vi "RPiReceive.vi"   [LabVIEW 2013]
uses:
  VisionData.ctl
types:
  T1 = typedef "VisionData.ctl" = cluster{"Total":u8, "Timestamp":u32, "Horizontal":u8, "Vertical":u8, "Left Hot":bool, "Right Hot":bool}
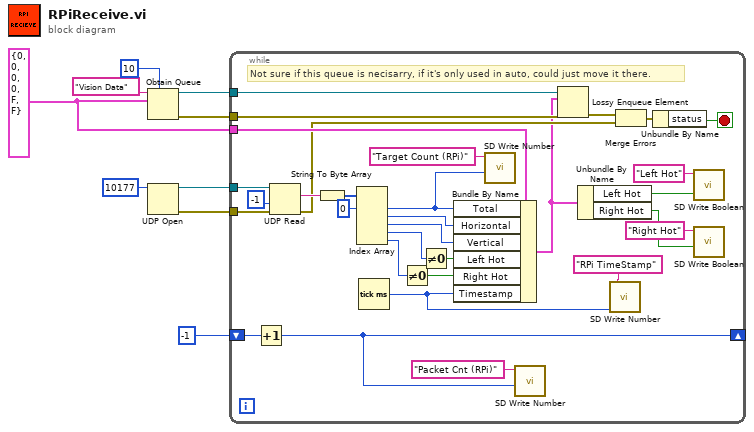
[diagram p0: block diagram]
diagram:
  w7 = T1 {"Total"=0, "Timestamp"=0, "Horizontal"=0, "Vertical"=0, "Left Hot"=FALSE, "Right Hot"=FALSE}
  n1 = Obtain Queue(max queue size (-1, unlimited)=10, name (unnamed)="Vision Data", element data type=w7) -> (queue out=w4:refnum<queue>, error out=w8:errorcluster)  [unwired: 2 in, 1 out]
  n2 = UDP Open(11:u16 10177 ("port")) -> (port=w2:refnum<k16>, 0:w3:errorcluster)  [unwired: 4 in, 1 out]
  n3 = while {
    tunnel: w2 -> [w40]
    tunnel: w3 -> [w39]
    tunnel: w4 -> [w35]
    tunnel: w7 -> [w34]
    tunnel: w8 -> [w33]
    shift-right: [w25] -> _
    shift-left: -1 -> [w24]
    stop <- w29 stop-if-true
    # "Not sure if this queue is necisarry, if it's only used in auto, could just move it there."
    n4 = Increment(x=w24) -> (x+1=w25:i32)
    n5 = UDP Read(connection ID=w40, timeout ms (25000)=-1, 8:w39) -> (data out=w37:string, error out=w31:errorcluster)  [unwired: 1 in, 3 out]
    n6 = String To Byte Array(string=w37) -> (unsigned byte array=w23:u8[])
    n7 = Index Array(array=w23, index #1=0 ("index")) -> (element #1=w15:u8, element #2=w22:u8, element #3=w21:u8, element #4=w18:u8, element #5=w16:u8)  [unwired: 4 in]
    n8 = Tick Count (ms)() -> (millisecond timer value=w20:u32)
    n9 = Not Equal To 0?(x=w16) -> (x != 0?=w17:bool)
    n10 = Not Equal To 0?(x=w18) -> (x != 0?=w19:bool)
    n11 = Bundle By Name(cluster=w34, "Total"=w15, "Horizontal"=w22, "Vertical"=w21, "Left Hot"=w19, "Right Hot"=w17, "Timestamp"=w20) -> (w14:T1)
    n12 = call <vilib>:"SD Write Number.vi"("Numeric"=w15, "Name"="Target Count (RPi)") -> ()  [unwired: 8 in, 2 out]
    n13 = call <vilib>:"SD Write Number.vi"("Numeric"=w25, "Name"="Packet Cnt (RPi)") -> ()  [unwired: 8 in, 2 out]
    n14 = Lossy Enqueue Element(queue=w35, element=w14, error in (no error)=w33) -> (error out=w32:errorcluster)  [unwired: 3 out]
    n15 = Unbundle By Name(w14) -> ("Left Hot"=w13:bool, "Right Hot"=w12:bool)
    n16 = call <vilib>:"SD Write Number.vi"("Numeric"=w20, "Name"="RPi TimeStamp") -> ()  [unwired: 8 in, 2 out]
    n17 = Merge Errors(w32, w31) -> (w30:errorcluster)
    n18 = Unbundle By Name(w30) -> ("status"=w29:bool)
    n19 = call <vilib>:"SD Write Boolean.vi"("Boolean"=w13, "Name"="Left Hot") -> ()  [unwired: 8 in, 2 out]
    n20 = call <vilib>:"SD Write Boolean.vi"("Boolean"=w12, "Name"="Right Hot") -> ()  [unwired: 8 in, 2 out]
  }
